vi "Untitled 2 (SubVI).vi"(1 "Numeric":u8) -> (0 "Cluster":T1 {"E" scale=0.0..1.0 scale format="%b"; "D" scale=0.0..1.0 scale format="%b"; "C" scale=0.0..1.0 scale format="%b"; "G" scale=0.0..1.0 scale format="%b"; "B" scale=0.0..1.0 scale format="%b"; "A" scale=0.0..1.0 scale format="%b"; "F" scale=0.0..1.0 scale format="%b"})   [LabVIEW 2022 SP3]
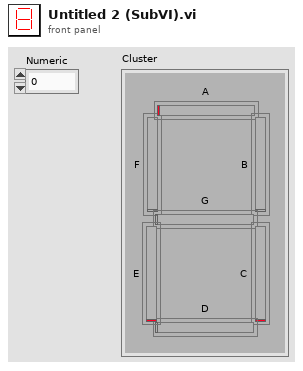
[diagram p1: front panel]
types:
  T1 = cluster{"F":u8, "A":u8, "B":u8, "G":u8, "C":u8, "D":u8, "E":u8}
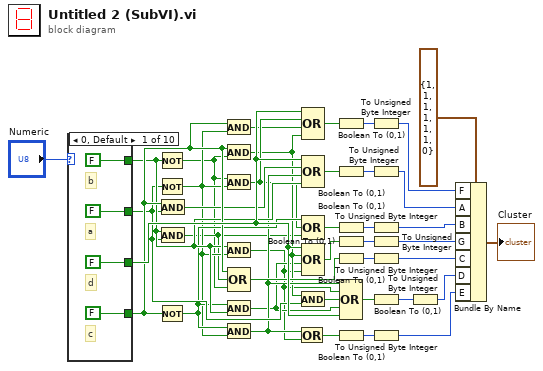
[diagram p0: block diagram]
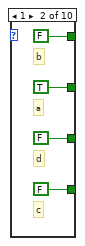
[diagram p2: hidden frame]
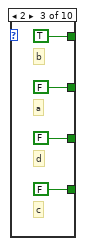
[diagram p3: hidden frame]
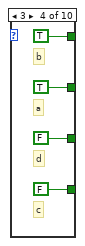
[diagram p4: hidden frame]
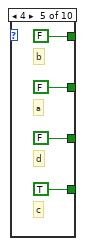
[diagram p5: hidden frame]
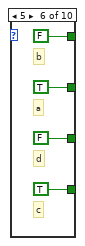
[diagram p6: hidden frame]
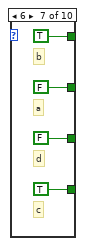
[diagram p7: hidden frame]
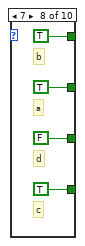
[diagram p8: hidden frame]
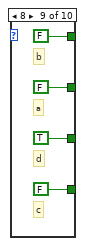
[diagram p9: hidden frame]
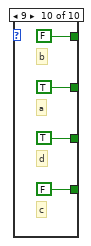
[diagram p10: hidden frame]
diagram:
  n1 = case shown="0, Default" "Numeric" {
    tunnel: [FALSE TRUE FALSE TRUE FALSE TRUE FALSE TRUE FALSE TRUE] -> w28
    tunnel: [FALSE FALSE TRUE TRUE FALSE FALSE TRUE TRUE FALSE FALSE] -> w29
    tunnel: [FALSE FALSE FALSE FALSE TRUE TRUE TRUE TRUE FALSE FALSE] -> w30
    tunnel: [FALSE FALSE FALSE FALSE FALSE FALSE FALSE FALSE TRUE TRUE] -> w31
    frame 0, Default {
      # "d"
      # "c"
      # "b"
      # "a"
    }
    frame 1 {
      # "d"
      # "c"
      # "b"
      # "a"
    }
    frame 2 {
      # "d"
      # "c"
      # "b"
      # "a"
    }
    frame 3 {
      # "d"
      # "c"
      # "b"
      # "a"
    }
    frame 4 {
      # "d"
      # "c"
      # "b"
      # "a"
    }
    frame 5 {
      # "d"
      # "c"
      # "b"
      # "a"
    }
    frame 6 {
      # "d"
      # "c"
      # "b"
      # "a"
    }
    frame 7 {
      # "d"
      # "c"
      # "b"
      # "a"
    }
    frame 8 {
      # "d"
      # "c"
      # "b"
      # "a"
    }
    frame 9 {
      # "d"
      # "c"
      # "b"
      # "a"
    }
  }
  n2 = Not(x=w29) -> (.not. x?=w1:bool)
  n3 = Not(x=w28) -> (.not. x?=w7:bool)
  n4 = Not(x=w30) -> (.not. x?=w10:bool)
  n5 = And(x=w30, y=w28) -> (x .and. y?=w12:bool)
  n6 = And(x=w29, y=w28) -> (x .and. y?=w2:bool)
  n7 = And(x=w30, y=w7) -> (x .and. y?=w6:bool)
  n8 = And(x=w30, y=w1) -> (x .and. y?=w5:bool)
  n9 = And(x=w1, y=w7) -> (x .and. y?=w8:bool)
  n10 = And(x=w29, y=w7) -> (x .and. y?=w3:bool)
  n11 = And(x=w10, y=w29) -> (x .and. y?=w4:bool)
  n12 = And(x=w10, y=w7) -> (x .and. y?=w9:bool)
  n13 = Compound Arithmetic op=OR(w30, w2, w1) -> (w17:bool)
  n14 = Or(x=w9, y=w3) -> (x .or. y?=w15:bool)
  n15 = And(x=w5, y=w28) -> (x .and. y?=w11:bool)
  n16 = Compound Arithmetic op=OR(w31, w8, w6, w5) -> (w14:bool)
  n17 = Compound Arithmetic op=OR(w31, w12, w9, w29) -> (w18:bool)
  n18 = Compound Arithmetic op=OR(w10, w8, w2) -> (w21:bool)
  n19 = Compound Arithmetic op=OR(w31, w5, w4, w3) -> (w13:bool)
  n20 = Boolean To (0,1)(Boolean=w14) -> (0, 1=w25:i16)
  n21 = Boolean To (0,1)(Boolean=w18) -> (0, 1=w19:i16)
  n22 = Boolean To (0,1)(Boolean=w21) -> (0, 1=w20:i16)
  n23 = Boolean To (0,1)(Boolean=w13) -> (0, 1=w26:i16)
  n24 = Boolean To (0,1)(Boolean=w17) -> (0, 1=w22:i16)
  n25 = Boolean To (0,1)(Boolean=w15) -> (0, 1=w24:i16)
  n26 = Compound Arithmetic op=OR(w9, w3, w11, w4, w31) -> (w16:bool)
  n27 = To Unsigned Byte Integer(number=w25) -> (unsigned 8bit integer=w34:u8)
  n28 = To Unsigned Byte Integer(number=w19) -> (unsigned 8bit integer=w33:u8)
  n29 = To Unsigned Byte Integer(number=w20) -> (unsigned 8bit integer=w38:u8)
  n30 = To Unsigned Byte Integer(number=w26) -> (unsigned 8bit integer=w36:u8)
  n31 = To Unsigned Byte Integer(number=w22) -> (unsigned 8bit integer=w39:u8)
  n32 = Boolean To (0,1)(Boolean=w16) -> (0, 1=w23:i16)
  n33 = To Unsigned Byte Integer(number=w24) -> (unsigned 8bit integer=w35:u8)
  n34 = To Unsigned Byte Integer(number=w23) -> (unsigned 8bit integer=w37:u8)
  n35 = Bundle By Name(cluster=T1 {"F"=1, "A"=1, "B"=1, "G"=1, "C"=1, "D"=1, "E"=0} ("Cluster"), "F"=w34, "A"=w33, "B"=w38, "G"=w36, "C"=w39, "D"=w37, "E"=w35) -> (→"Cluster":T1)
